vi "BenchC2_DEV_v15_5.vi"() -> ()   [LabVIEW 2016]
uses:
  BERTTA/x64/Debug/BERTTA.dll
panel:
  out "Started:":string
  in  "SHUTDOWN":bool
  in  "MASTER CONTROL":bool
  in  "Tab Control":T1(tab)
  out "Output File":path caption="selected path"
  in  "Browse folder":path=path "C:/Users/shresplab/Desktop" caption="start path"
  in  "Read Seq":bool
  in  "Save Seq":bool
  in  "Configuration file":path caption="Filename"
  in  "OK Button 2":bool
  out "Boolean":bool
  in  "User (initials)":string
  in  "Project name":string
  in  "Description":string
  out "Led11 12":bool
  out "Led11 11":bool
  out "PUMP1":bool
  out "Target amount":dbl format="Target amount:        %#_g"
  out "Scale weight":dbl format="Scale weight:     %#_4g"
  out "Amount now":dbl format="Amount now:      %#_4g"
  out "Flow rate":dbl format="Flow rate:                   %#_4g"
  out "Time to target":dbl format="Time to target:     %<%H:%M:%S>t"
  out "Current step":dbl format="Current step:              %#_g"
  out "Target":dbl format="Target:                %#_4g"
  out "Amount now":dbl format="Amount now:    %#_4g"
  out "Amount now":dbl
  out "Target":dbl
  out "Current step":dbl
  out "Time to target":dbl format="%<%H:%M:%S>t"
  out "Flow rate":dbl
  out "Amount now":dbl
  out "Scale weight":dbl
  out "Target amount":dbl
  out "PUMP2":bool
  out "Sensor OK 6":bool
  out "Sensor OK 5":bool
  out "Sensor OK 4":bool
  out "Sensor OK 3":bool
  in  "OK Button":bool
  in  "Add comment":string
  out "Tr":dbl format="Tr:              %#_4g"
  out "Tj in":dbl format="Tj in:        %#_4g"
  out "Tj out":dbl format="Tj out:        %#_4g"
  out "T set":dbl format="T set:          %#_g"
  out "Current step":i32 format="Current step:  %.0f"
  out "RPM":dbl format="RPM:          %#_g"
  out "Torque 2":dbl format="Torque:      %#_g"
  out "PUMP3":bool
  out "Target amount":dbl
  out "Scale weight":dbl
  out "Amount now":dbl
  out "Flow rate":dbl
  out "Time to target":dbl format="%<%H:%M:%S>t"
  out "Current step":dbl
  out "Target":dbl
  out "Amount now":dbl
  out "Waveform Chart 5":dynamicdata(graph)
  out "Waveform Chart 6":dynamicdata(graph)
  out "Waveform Chart 7":dynamicdata(graph)
  out "Led11 10":bool
  out "T external 3":dbl format="T (S2):       %#_4g"
  out "Table":string[][](table)=[["14.8.2017 18.06.59", "0,000000", "417,670000", "-0,150000", "1,000000", "22,220000", "23,366837", "23,574959", "23,985852", "23,690000", "240,000000", "4,000000", "0,000000", "397,000000", "-397,000000", "1,000000"], ["14.8.2017 18.07.06", "0,000000", "417,640000", "-0,120000", "1,000000", "22,220000", "23,763115", "23,906257", "23,985694", "23,680000", "240,000000", "4,000000", "0,000000", "397,000000", "-397,000000", "1,000000"], ["14.8.2017 18.07.13", "0,000000", "417,640000", "-0,120000", "1,000000", "22,220000", "23,965922", "24,013440", "23,984906", "23,670000", "240,000000", "4,100000", "3,000000", "397,000000", "-397,000000", "1,000000"], ["14.8.2017 18.07.21", "0,000000", "417,640000", "-0,120000", "1,000000", "22,220000", "23,943860", "23,900110", "23,987113", "23,670000", "240,000000", "4,000000", "0,000000", "397,000000", "-397,000000", "1,000000"], ["14.8.2017 18.07.28", "0,000000", "417,640000", "-0,120000", "1,000000", "22,220000", "23,736328", "23,600018", "23,989004", "23,660000", "240,000000", "4,000000", "0,000000", "397,000000", "-397,000000", "1,000000"], ["14.8.2017 18.07.36", "0,000000", "417,640000", "-0,120000", "1,000000", "22,220000", "23,480910", "23,324538", "23,991053", "23,660000", "240,000000", "4,000000", "0,000000", "397,000000", "-397,000000", "1,000000"], ["14.8.2017 18.07.43", "0,000000", "417,640000", "-0,120000", "2,000000", "22,220000", "23,195579", "23,008270", "23,999093", "23,650000", "240,000000", "4,000000", "0,000000", "397,000000", "-397,000000", "1,000000"], ["14.8.2017 18.07.51", "0,000000", "417,650000", "-417,650000", "1,000000", "22,220000", "22,862541", "22,649021", "24,003979", "23,650000", "240,000000", "4,000000", "0,000000", "397,000000", "-397,000000", "2,000000"], ["14.8.2017 18.07.58", "0,000000", "417,640000", "0,010000", "1,000000", "22,220000", "22,541353", "22,354878", "24,005398", "23,650000", "240,000000", "4,000000", "0,000000", "397,000000", "-397,000000", "1,000000"], ["14.8.2017 18.08.06", "0,000000", "417,640000", "0,010000", "1,000000", "22,220000", "22,347931", "22,253738", "24,007605", "23,640000", "240,000000", "4,100000", "0,000000", "397,000000", "-397,000000", "1,000000"], ["14.8.2017 18.08.13", "0,000000", "417,640000", "0,010000", "1,000000", "22,220000", "22,329030", "22,302102", "24,006028", "23,640000", "240,000000", "4,000000", "0,000000", "395,820000", "-395,820000", "1,000000"], ["14.8.2017 18.08.20", "0,000000", "417,640000", "0,010000", "1,000000", "22,220000", "22,466849", "22,511320", "24,002403", "23,630000", "240,000000", "4,000000", "0,000000", "395,830000", "-0,010000", "1,000000"], ["14.8.2017 18.08.28", "0,000000", "417,640000", "0,010000", "1,000000", "22,220000", "22,707062", "22,835101", "24,000984", "23,620000", "240,000000", "4,000000", "0,000000", "395,830000", "-0,010000", "1,000000"], ["14.8.2017 18.08.35", "0,000000", "417,640000", "0,010000", "1,000000", "22,220000", "23,054104", "23,232979", "24,001299", "23,600000", "240,000000", "4,000000", "0,000000", "395,830000", "-0,010000", "1,000000"], ["14.8.2017 18.08.43", "0,000000", "417,640000", "0,010000", "1,000000", "22,220000", "23,412371", "23,522793", "24,002560", "23,590000", "240,000000", "4,000000", "0,000000", "395,820000", "0,000000", "1,000000"], ["14.8.2017 18.08.51", "0,000000", "417,640000", "0,010000", "1,000000", "22,220000", "23,596247", "23,656125", "24,003821", "23,580000", "240,000000", "4,000000", "0,000000", "395,820000", "0,000000", "1,000000"]]
  out "LED_5":bool
  out "LED_4":bool
  in  "PAUSE/RUN 4":bool
  in  "TEMP RAMP":dbl[][](array[numeric])
  out "LED_3":bool
  out "LED_2":bool
  out "LED_1":bool
  out "LED_MANUAL":bool
  in  "Reset 6":bool
  in  "Manual/Ramp":bool=TRUE
  in  "Sensor selector":bool=TRUE
  in  "Tr/Tj mode selector":bool=TRUE
  out "LED STOP":bool
  in  "Failsafe":dbl=20.0 format="Failsafe temperature:            %#_g"
  out "Current temp":dbl format="Current temperature S1:       %#_4g"
  out "Sensor OK":bool
  out "T external 2":dbl format="Current temperature S2:       %#_4g"
  in  "OK Button 3":bool
  out "Waveform Chart":dynamicdata(graph)
  in  "X scale":i64(slide)=50 scale=0.0..100.0
  in  "PAUSE/RUN 9":bool=TRUE
  in  "PAUSE/RUN 8":bool=TRUE
  in  "PAUSE/RUN 7":bool=TRUE
  out "Led11 7":bool
  out "Led11 6":bool
  out "Led11 7":bool
  out "Led11 6":bool
  out "Led5 7":bool
  out "Led4 6":bool
  out "Waveform Chart 18":dynamicdata(graph)
  in  "PAUSE/RUN 3":bool
  in  "Tube select 3":u32(ring) items=["Big tube", "Double big tube", "Medium tube", "Small tube"]
  in  "Reset 8":bool
  out "Led11 9":bool
  in  "?":bool
  in  "Grams / min 3":dbl
  out "RPM 3":dbl format="%_4f"
  out "Flow rate (g/min) 3":dbl
  out "Scale reading 3":dbl
  out "Step amount now 3":dbl
  out "Total amount now 3":dbl
  out "Elapsed / step 3":dbl format="%<%H:%M:%S>t"
  out "Time to target 3":dbl format="%<%H:%M:%S>t"
  out "Led5 5":bool
  out "Led4 5":bool
  out "Led3 5":bool
  out "Led2 5":bool
  out "Led1 5":bool
  in  "PumpSeq 6":dbl[][](array[numeric])=[[0.0, 0.0, 0.0, 0.0, 0.0, 0.0, 0.0, 0.0, 0.0, 0.0], [0.0, 0.0, 0.0, 0.0, 0.0, 0.0, 0.0, 0.0, 0.0, 0.0], [0.0, 0.0, 0.0, 0.0, 0.0, 0.0, 0.0, 0.0, 0.0, 0.0], [0.0, 0.0, 0.0, 0.0, 0.0, 0.0, 0.0, 0.0, 0.0, 0.0], [0.0, 0.0, 0.0, 0.0, 0.0, 0.0, 0.0, 0.0, 0.0, 0.0], [0.0, 0.0, 0.0, 0.0, 0.0, 0.0, 0.0, 0.0, 0.0, 0.0], [0.0, 0.0, 0.0, 0.0, 0.0, 0.0, 0.0, 0.0, 0.0, 0.0], [0.0, 0.0, 0.0, 0.0, 0.0, 0.0, 0.0, 0.0, 0.0, 0.0], [0.0, 0.0, 0.0, 0.0, 0.0, 0.0, 0.0, 0.0, 0.0, 0.0], [0.0, 0.0, 0.0, 0.0, 0.0, 0.0, 0.0, 0.0, 0.0, 0.0]]
  out "Led11 8":bool
  in  "PAUSE/RUN 2":bool
  in  "Tube select 2":u32(ring) items=["Big tube", "Double big tube", "Medium tube", "Small tube"]
  out "Led11 7":bool
  in  "?":bool
  in  "Grams / min 2":dbl
  out "RPM 2":dbl format="%_4f"
  out "Flow rate (g/min) 2":dbl
  out "Scale reading 2":dbl
  out "Step amount now 2":dbl
  out "Total amount now 2":dbl
  out "Elapsed / step 2":dbl format="%<%H:%M:%S>t"
  out "Time to target 2":dbl format="%<%H:%M:%S>t"
  out "Led5 4":bool
  out "Led4 4":bool
  out "Led3 4":bool
  out "Led2 4":bool
  out "Led1 4":bool
  in  "PumpSeq 5":dbl[][](array[numeric])=[[0.0, 0.0, 0.0, 0.0, 0.0, 0.0, 0.0, 0.0, 0.0, 0.0], [0.0, 0.0, 0.0, 0.0, 0.0, 0.0, 0.0, 0.0, 0.0, 0.0], [0.0, 0.0, 0.0, 0.0, 0.0, 0.0, 0.0, 0.0, 0.0, 0.0], [0.0, 0.0, 0.0, 0.0, 0.0, 0.0, 0.0, 0.0, 0.0, 0.0], [0.0, 0.0, 0.0, 0.0, 0.0, 0.0, 0.0, 0.0, 0.0, 0.0], [0.0, 0.0, 0.0, 0.0, 0.0, 0.0, 0.0, 0.0, 0.0, 0.0], [0.0, 0.0, 0.0, 0.0, 0.0, 0.0, 0.0, 0.0, 0.0, 0.0], [0.0, 0.0, 0.0, 0.0, 0.0, 0.0, 0.0, 0.0, 0.0, 0.0], [0.0, 0.0, 0.0, 0.0, 0.0, 0.0, 0.0, 0.0, 0.0, 0.0], [0.0, 0.0, 0.0, 0.0, 0.0, 0.0, 0.0, 0.0, 0.0, 0.0]]
  out "Led11 6":bool
  in  "Reset 7":bool
  in  "PAUSE/RUN":bool
  in  "Tube select":u32(ring) items=["Big tube", "Double big tube", "Medium tube", "Small tube"]
  out "Led11 5":bool
  out "RPM":dbl format="RPM                      %_4f"
  out "Flow rate (g/min)":dbl format="Flow rate               %#_g"
  out "Scale reading":dbl format="Scale reading       %#_g"
  out "Step amount now":dbl format="Step amount       %#_g"
  out "Total amount now":dbl format="Total amount      %#_g"
  out "Elapsed / step":dbl format="Elapsed / step      %<%H:%M:%S>t"
  out "Time to target":dbl format="Time to target     %<%H:%M:%S>t"
  out "Led5 3":bool
  out "Led4 3":bool
  out "Led3 3":bool
  out "Led2 3":bool
  out "Led1 3":bool
  in  "PumpSeq 4":dbl[][](array[numeric])=[[0.0, 0.0, 0.0, 0.0, 0.0, 0.0, 0.0, 0.0, 0.0, 0.0], [0.0, 0.0, 0.0, 0.0, 0.0, 0.0, 0.0, 0.0, 0.0, 0.0], [0.0, 0.0, 0.0, 0.0, 0.0, 0.0, 0.0, 0.0, 0.0, 0.0], [0.0, 0.0, 0.0, 0.0, 0.0, 0.0, 0.0, 0.0, 0.0, 0.0], [0.0, 0.0, 0.0, 0.0, 0.0, 0.0, 0.0, 0.0, 0.0, 0.0], [0.0, 0.0, 0.0, 0.0, 0.0, 0.0, 0.0, 0.0, 0.0, 0.0], [0.0, 0.0, 0.0, 0.0, 0.0, 0.0, 0.0, 0.0, 0.0, 0.0], [0.0, 0.0, 0.0, 0.0, 0.0, 0.0, 0.0, 0.0, 0.0, 0.0], [0.0, 0.0, 0.0, 0.0, 0.0, 0.0, 0.0, 0.0, 0.0, 0.0], [0.0, 0.0, 0.0, 0.0, 0.0, 0.0, 0.0, 0.0, 0.0, 0.0]]
  in  "?":bool
  in  "Grams / min":dbl format="Manual g/min:  %#_g"
  out "Led11 4":bool
  in  "Reset 5":bool
  in  "OK Button 4":bool
  out "Waveform Chart 16":dynamicdata(graph)
  in  "OK Button 5":bool
  out "Waveform Chart 17":dynamicdata(graph)
  in  "OK Button 6":bool
  in  "PAUSE/RUN 5":bool
  in  "?":bool
  in  "Scale port":dbl=5.0
  out "Waveform Chart 15":dynamicdata(graph)
  in  "OK Button 8":bool
  in  "PAUSE/RUN 6":bool
  in  "Set RPM":i32
  in  "Remote / Manual":bool
  out "RPM":dbl
  out "Torque":dbl
  out "Waveform Chart 4":dynamicdata(graph)
  in  "OK Button 7":bool
  in  "CDAQ Temp Control":tag="cDAQ9188XT-1C3BF12Mod1"
  in  "CDAQ PAM Control":tag="cDAQ9188XT-1C3BF12Mod1"
  in  "PORT PUMP2":i32 format="PUMP 2 PORT:  %.0f"
  in  "PORT PUMP3":i32 format="PUMP 3 PORT:  %.0f"
  in  "PORT PUMP1":i32 format="PUMP 1 PORT:  %.0f"
  in  "Save PortDev":bool
  in  "LAUDA":i32 format="LAUDA PORT:  %.0f"
  in  "HEIDOLPH":i32 format="HEIDOLPH PORT:  %.0f"
  in  "SCALE1":i32 format="SCALE 1 PORT:  %.0f"
  in  "SCALE2":i32 format="SCALE 2 PORT:  %.0f"
  in  "SCALE 3":i32 format="SCALE 3 PORT:  %.0f"
  # "PUMP & SCALE 1"
  # "PUMP & SCALE 2"
  # "PUMP & SCALE 3"
  # "STEP"
  # "STEP"
  # "STEP"
  # "TOTAL"
  # "TOTAL"
  # "TOTAL"
  # "Temperature sensor:"
  # "Manual control:"
  # "MANUAL"
  # "RAMP"
  # "Temp Target       Time Target          Wait Time"
  # "STOP"
  # "g              min"
  # "g              min"
  # "g              min"
  # "PAM control"
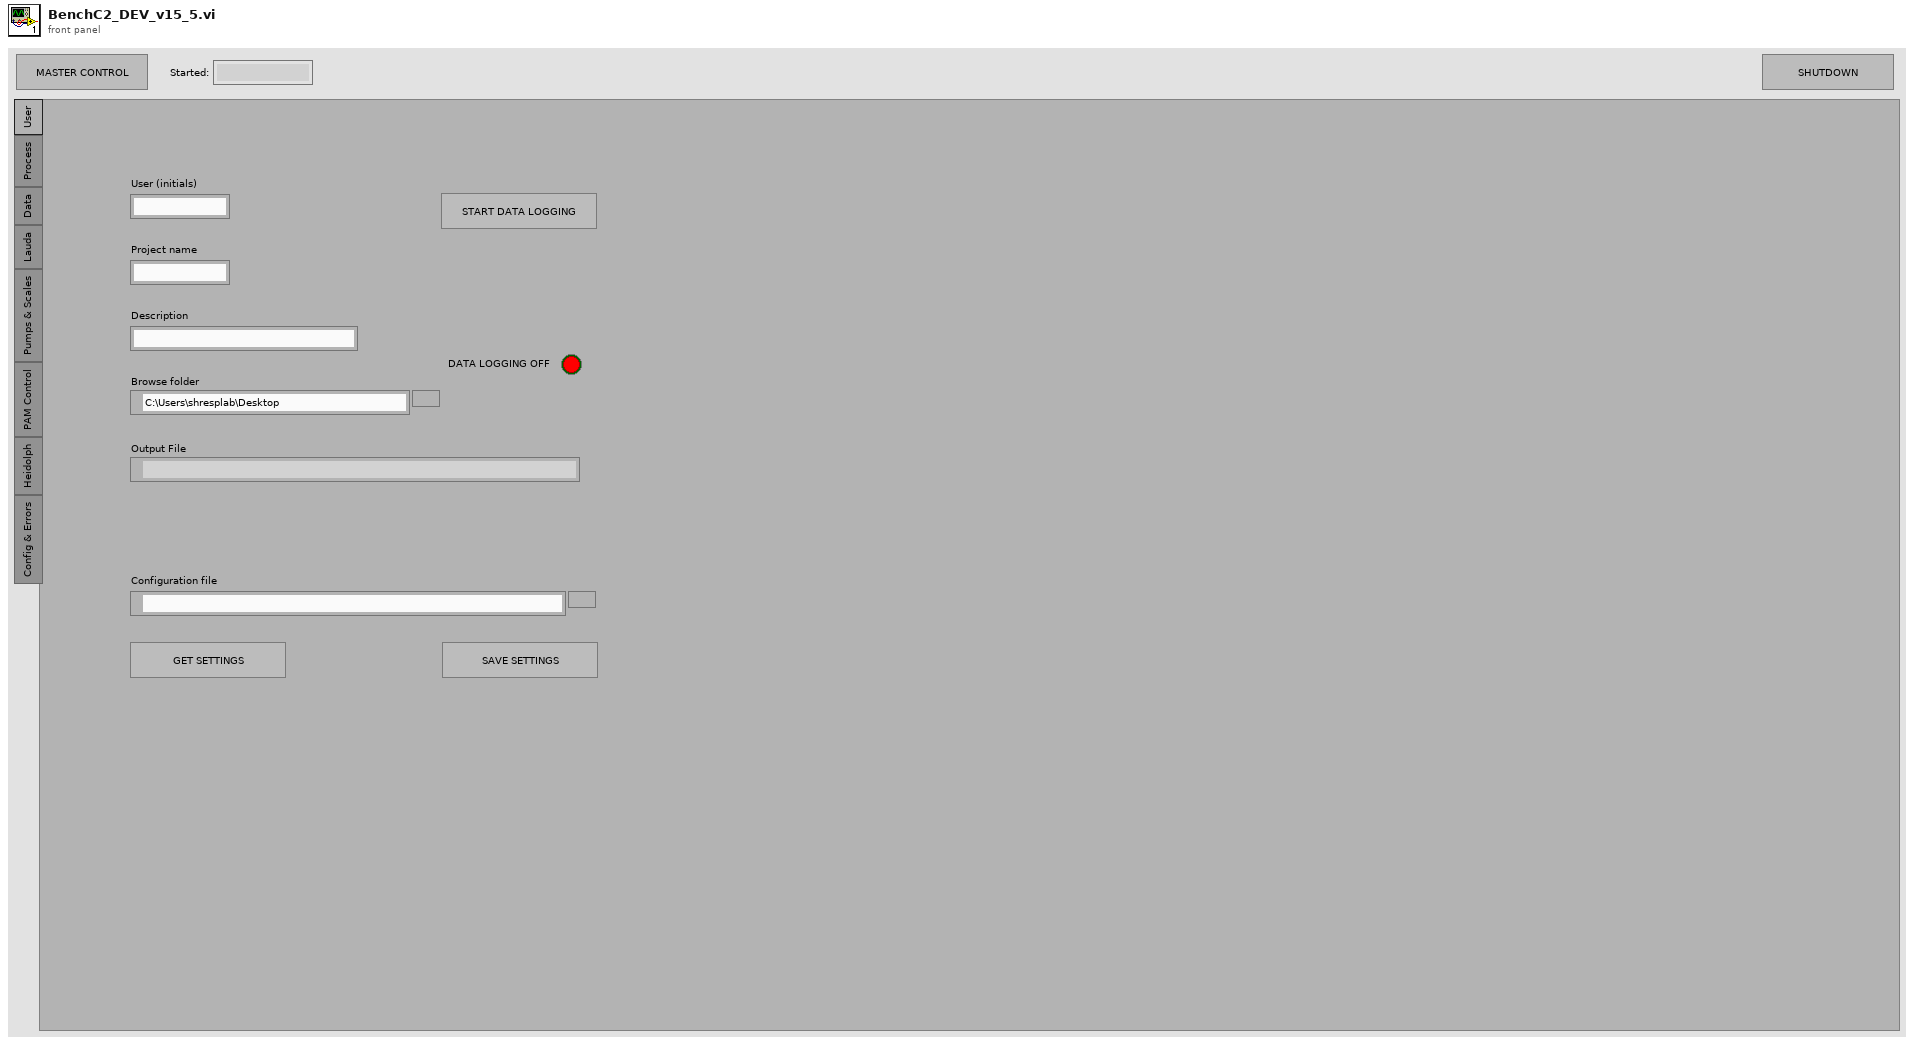
[diagram p1: front panel]
types:
  T1 = enum32{"User", "Process", "Data", "Lauda", "Pumps & Scales", "PAM Control", "Heidolph", "Config & Errors"}
diagram:
  n1 = while {
    i -> [w211]
    stop <- FALSE stop-if-true
    w105 = i64 1000 ("y")
    # "SCALE & PUMP 3"
    n2 = Boolean To (0,1)(Boolean="PAUSE/RUN 7") -> (0, 1=w3:i16)
    n3 = Boolean To (0,1)(Boolean="PAUSE/RUN 8") -> (0, 1=w2:i16)
    n4 = Boolean To (0,1)(Boolean="PAUSE/RUN 9") -> (0, 1=w1:i16)
    n5 = And(x="PAUSE/RUN 6", y="MASTER CONTROL") -> (x .and. y?=w94:bool)
    n6 = feedback #1() -> (w110:dbl[][])  [unwired: 1 in]
    n7 = Select(t="TEMP RAMP", s="Reset 6", f=w110) -> (s? t:f=w111:dbl[][])
    n8 = feedback-in #1(w111) -> ()
    n9 = Initialize Array(0.0 ("element"), 5 ("dimension size"), 3 ("dimension size")) -> (w154:dbl[][])
    n10 = Select(t="Set RPM", s=w94, f=10) -> (s? t:f=w97:i32)
    n11 = Not(x="MASTER CONTROL") -> (.not. x?=w260:bool)
    n12 = Replace Array Subset(array=w154, new element=w110, index (row)=0, index (col)=0 ("disabled index (col)")) -> (w128:dbl[][])
    n13 = control-ref of="This VI"() -> (w90:refnum<vi>)
    n14 = Multiply(x="X scale", y=w105) -> (x*y=w106:i64)
    n15 = Boolean To (0,1)(Boolean=w260) -> (0, 1=w261:i16)
    n16 = Add(x=w106, y=w105) -> (x+y=w101:i64)
    n17 = for {
      N: w261 -> [_]
      n18 = Get Date/Time String(want seconds? (F)=TRUE) -> (time string=→"Started:":string)  [unwired: 2 in, 1 out]
    }
    n19 = feedback #2() -> (w104:i64)  [unwired: 1 in]
    n20 = feedback-in #2(w101) -> ()
    n21 = Boolean To (0,1)(Boolean="Sensor selector") -> (0, 1=w136:i16)
    n22 = Boolean To (0,1)(Boolean="SHUTDOWN") -> (0, 1=w88:i16)
    n23 = call "shutdown sequence.vi"("SHUTDOWN"="SHUTDOWN", "VI in"=w90) -> ()  [unwired: 10 in]
    n24 = Not Equal?(x=w104, y=w101) -> (x != y?=w103:bool)
    n25 = property on="Waveform Chart" class="WFChart (strict)"() -> ("History Data"=w108:dynamicdata[])  [unwired: 2 in, 2 out]
    n26 = Boolean To (0,1)(Boolean=w103) -> (0, 1=w100:i16)
    n27 = Array Size(array=w108) -> (size(s)=w102:i32)
    n28 = Boolean To (0,1)(Boolean="SHUTDOWN") -> (0, 1=w91:i16)
    n29 = Boolean To (0,1)(Boolean="Tr/Tj mode selector") -> (0, 1=w148:i16)
    n30 = formula code="int SensorLED1 = 0, SensorLED0 = 0, ModeLED1 = 0, ModeLED0 = 0;\nif(Sensor==1) SensorLED1 = 1;\nif(Sensor==0) SensorLED0 = 1;\nif(Tr_Tj==1) ModeLED1 = 1;\nif(Tr_Tj==0) ModeLED0 = 1;"("Tr_Tj"=w148, "Sensor"=w136) -> ("SensorLED1"=w146:i32, "SensorLED0"=w144:i32, "ModeLED1"=w129:i32, "ModeLED0"=w139:i32)
    n31 = Equal?(x=w146, y=1.0) -> (x = y?=→"Sensor OK 3":bool)
    n32 = Equal?(x=w144, y=1.0) -> (x = y?=→"Sensor OK 4":bool)
    n33 = for {
      N: w100 -> [_]
      tunnel: w102 -> [w268]
      tunnel: w101 -> [w267]
      n34 = Add(x=w268, y=w267) -> (x+y=w266:i64)
      n35 = property on="Waveform Chart" class="WFChart (strict)"("XScale.Maximum"=w266) -> ()  [unwired: 2 in, 2 out]
    }
    n36 = call "MReadRS232_2.vi"("port1"="LAUDA", "dev1"=1, "enable5"=w3, "port2"="LAUDA", "dev2"=2, "port3"="HEIDOLPH", "enable7"=w1, "enable8"=0, "dev7"=5, "dev8"=0, "port7"="SCALE 3", "port8"=0, "dev5"=5, "enable6"=w2, "port5"="SCALE1", "dev4"=4, "dev6"=5, "port6"="SCALE2", "port4"="HEIDOLPH", "dev3"=3) -> ("params"=w27:dbl[])  [unwired: 6 in, 1 out]
    n37 = call "HEI_CTRL.vi"("shutdown"=w91, "Set RPM"=w97, "Remote / Manual"="Remote / Manual", "port3"="HEIDOLPH") -> ()  [unwired: 8 in]
    n38 = And(x="MASTER CONTROL", y="PAUSE/RUN 4") -> (x .and. y?=w170:bool)
    n39 = Index Array(array=w128, index (col)=2 ("disabled index (col)")) -> (element=w158:dbl[])  [unwired: 1 in]
    n40 = Equal?(x=w129, y=1.0) -> (x = y?=→"Sensor OK 6":bool)
    n41 = Equal?(x=w139, y=1.0) -> (x = y?=→"Sensor OK 5":bool)
    n42 = Boolean To (0,1)(Boolean=w170) -> (0, 1=w169:i16)
    n43 = Boolean To (0,1)(Boolean="Manual/Ramp") -> (0, 1=w171:i16)
    n44 = Boolean To (0,1)(Boolean="Reset 6") -> (0, 1=w173:i16)
    n45 = Build Array("LAUDA", "HEIDOLPH", "SCALE1", "SCALE2", "SCALE 3", "PORT PUMP1", "PORT PUMP2", "PORT PUMP3") -> (w115:i32[])
    n46 = Index Array(array=w128, index (col)=1 ("disabled index (col)")) -> (element=w160:dbl[])  [unwired: 1 in]
    n47 = Index Array(array=w128, index (col)=0 ("disabled index (col)")) -> (element=w161:dbl[])  [unwired: 1 in]
    n48 = call "LaudaDAQ.vi"("device name"="CDAQ Temp Control") -> (1:"Tj out"=→"Tj out":dbl, "data"=w248:dynamicdata, "Sensor OK"=→"Sensor OK":bool, 4:"Tj out"=→"Tj in":dbl, "T external 2"=w93:dbl)  [unwired: 5 in, 1 out]
    "T external 2" <- w93
    "T external 3" <- w93
    n49 = call "Ramp_Lauda_v3.vi"("manual"=w171, "Tr_Tj"=w148, "shutdown"=w88, "S1_S2"=w136, "Tr"=w27, "T_fail"="Failsafe", "enable"=w169, "time_set"=w160, "reset"=w173, "time_wait"=w158, "T_S2"=w93, "port"="LAUDA", "T_sp"=w161) -> ("LED_1"=→"LED_1":bool, "LED_manual"=→"LED_MANUAL":bool, "LED_2"=→"LED_2":bool, "step"=w126:dbl, "LED_stop"=→"LED STOP":bool, "LED_3"=→"LED_3":bool, "LED 4"=→"LED_4":bool, "LED 5"=→"LED_5":bool, "setpoint"=w123:dbl, "Tr_out"=w168:dbl, "T int"=w167:dbl)  [unwired: 2 in, 2 out]
    "Tr" <- w168
    "T set" <- w123
    "Current temp" <- w168
    n50 = Boolean To (0,1)(Boolean="Save PortDev") -> (0, 1=w214:i16)
    n51 = for {
      N: w214 -> [_]
      tunnel: w115 -> [w314]
      tunnel: "Save PortDev" -> [w315]
      n52 = call "Convert to Dynamic Data"("Array"=w314) -> ("Dynamic Data Type"=w313:dynamicdata)  [unwired: 3 in]
      n53 = call "Write To Measurement File3"("Signals"=w313, "Reset"=w315) -> ()  [unwired: 15 in, 3 out]
    }
    n54 = Add(x=w126, y=1.0) -> (x+y=→"Current step":dbl)
    n55 = Less?(x=w211, y=1.0) -> (x < y?=w209:bool)
    n56 = Index Array(array=w27, index=3) -> (element=w202:dbl)
    "RPM" <- w202
    "RPM" <- w202
    n57 = Index Array(array=w27, index=2) -> (element=w204:dbl)
    n58 = Boolean To (0,1)(Boolean=w209) -> (0, 1=w210:i16)
    n59 = Divide(x=w204, y=10.0) -> (x/y=w201:dbl)
    "Torque" <- w201
    "Torque 2" <- w201
    n60 = for {
      N: w210 -> [_]
      tunnel: w209 -> [w308]
      n61 = while {
        tunnel: [w311] -> w307
        tunnel: w308 -> [w309]
        stop <- w312 stop-if-true
        n62 = call "Read From Measurement File2"("Enable"=TRUE, "Reset"=w309) -> ("Signals"=w311:dynamicdata, "EOF?"=w312:bool)  [unwired: 4 in, 4 out]
      }
      n63 = call "Convert from Dynamic Data2"("Dynamic Data Type"=w307) -> ("Array"=w293:dbl[])  [unwired: 3 in]
      n64 = Index Array(array=w293, index=0) -> (element=w300:dbl)
      n65 = Index Array(array=w293, index=1) -> (element=w299:dbl)
      n66 = Index Array(array=w293, index=2) -> (element=w298:dbl)
      n67 = Index Array(array=w293, index=3) -> (element=w297:dbl)
      n68 = Index Array(array=w293, index=4) -> (element=w296:dbl)
      n69 = Index Array(array=w293, index=5) -> (element=w290:dbl)
      n70 = Index Array(array=w293, index=6) -> (element=w292:dbl)
      n71 = Index Array(array=w293, index=7) -> (element=w291:dbl)
      n72 = property on="LAUDA" class="DigNum (strict)"("Val(Sgnl)"=w300) -> ()  [unwired: 2 in, 2 out]
      n73 = property on="HEIDOLPH" class="DigNum (strict)"("Val(Sgnl)"=w299) -> ()  [unwired: 2 in, 2 out]
      n74 = property on="SCALE1" class="DigNum (strict)"("Val(Sgnl)"=w298) -> ()  [unwired: 2 in, 2 out]
      n75 = property on="SCALE2" class="DigNum (strict)"("Val(Sgnl)"=w297) -> ()  [unwired: 2 in, 2 out]
      n76 = property on="SCALE 3" class="DigNum (strict)"("Val(Sgnl)"=w296) -> ()  [unwired: 2 in, 2 out]
      n77 = property on="PORT PUMP2" class="DigNum (strict)"("Val(Sgnl)"=w292) -> ()  [unwired: 2 in, 2 out]
      n78 = property on="PORT PUMP3" class="DigNum (strict)"("Val(Sgnl)"=w291) -> ()  [unwired: 2 in, 2 out]
      n79 = property on="PORT PUMP1" class="DigNum (strict)"("Val(Sgnl)"=w290) -> ()  [unwired: 2 in, 2 out]
    }
    n80 = Merge Signals(w202, w201) -> (w200:dynamicdata)
    "Waveform Chart 4" <- w200
    "Waveform Chart 6" <- w200
    n81 = Boolean To (0,1)(Boolean="OK Button 3") -> (0, 1=w229:i16)
    n82 = for {
      N: w229 -> [_]
      n83 = property on="Waveform Chart" class="WFChart (strict)"("History Data"=dynamicdata[] []) -> ()  [unwired: 2 in, 2 out]
    }
    n84 = Merge Signals(w123, w168, w167, w248) -> (w249:dynamicdata)
    "Waveform Chart" <- w249
    "Waveform Chart 5" <- w249
    n85 = Boolean To (0,1)(Boolean="OK Button 4") -> (0, 1=w227:i16)
    n86 = for {
      N: w227 -> [_]
      n87 = property on="Waveform Chart 18" class="WFChart (strict)"("History Data"=dynamicdata[] []) -> ()  [unwired: 2 in, 2 out]
    }
    n88 = call "IsmaCTRL.vi"("FR_manual"="Grams / min", "tube selector"="Tube select", "Manual"="?", "Reset"="Reset 5", "Pause"="PAUSE/RUN", "Setpoint_W   /   Setpoint_T"="PumpSeq 4", "Enable"="MASTER CONTROL", "Scale"=w27) -> ("Boolean 9"=→"Led11 5" →"Led11 10":bool, "Boolean"=→"Led1 3":bool, "Boolean 2"=→"Led2 3":bool, "Total target"=→"Target":dbl, "Boolean 3"=→"Led3 3":bool, "Boolean 4"=→"Led4 3":bool, "lastAmount"=→"Step amount now":dbl, "step"=→"Current step":dbl, "Boolean 5"=→"Led5 3":bool, "Boolean 6"=→"Led4 6":bool, "Boolean 7"=→"Led5 7":bool, "FR"=w70:dbl, "RPM"=w62:dbl, "Weight"=w66:dbl, "elapsed"=→"Elapsed / step":dbl, "time_to_target"=→"Time to target" →"Time to target":dbl, "pumpCTRL"=w82:dbl, "Target_step"=→"Target amount":dbl, "Boolean 8"=w74:bool)  [unwired: 1 out]
    "Flow rate" <- w70
    "Scale weight" <- w66
    "Led11 4" <- w74
    "Scale reading" <- w66
    "Flow rate (g/min)" <- w70
    "RPM" <- w62
    n89 = Boolean To (0,1)(Boolean="OK Button 5") -> (0, 1=w134:i16)
    n90 = for {
      N: w134 -> [_]
      n91 = property on="Waveform Chart 16" class="WFChart (strict)"("History Data"=dynamicdata[] []) -> ()  [unwired: 2 in, 2 out]
    }
    n92 = Multiply(x=w66, y=-1.0 ("x")) -> (x*y=→"Amount now" →"Amount now" →"Total amount now":dbl)
    n93 = Greater?(x=w82, y=70.0) -> (0:→"PUMP1":bool)
    n94 = Boolean To (0,1)(Boolean="OK Button 6") -> (0, 1=w132:i16)
    n95 = And(x="PAUSE/RUN", y=w74) -> (x .and. y?=w190:bool)
    n96 = Merge Signals(w66, w70) -> (w135:dynamicdata)
    "Waveform Chart 18" <- w135
    n97 = for {
      N: w132 -> [_]
      n98 = property on="Waveform Chart 17" class="WFChart (strict)"("History Data"=dynamicdata[] []) -> ()  [unwired: 2 in, 2 out]
    }
    n99 = feedback #3() -> (w191:bool)  [unwired: 1 in]
    n100 = feedback-in #3(w190) -> ()
    n101 = Not Equal?(x=w191, y=w190) -> (x != y?=w189:bool)
    n102 = Boolean To (0,1)(Boolean=w189) -> (0, 1=w188:i16)
    n103 = for {
      N: w188 -> [_]
      n104 = property on="PAUSE/RUN" class="Bool (strict)"("Val(Sgnl)"=FALSE ("Value (Signaling)")) -> ()  [unwired: 2 in, 2 out]
    }
    n105 = Boolean To (0,1)(Boolean="OK Button 7") -> (0, 1=w225:i16)
    n106 = for {
      N: w225 -> [_]
      n107 = property on="Waveform Chart 4" class="WFChart (strict)"("History Data"=dynamicdata[] []) -> ()  [unwired: 2 in, 2 out]
    }
    n108 = Boolean To (0,1)(Boolean="OK Button 8") -> (0, 1=w197:i16)
    n109 = call "IsmaCTRL_2.vi"("FR_manual"="Grams / min 2", "tube selector"="Tube select 2", "Manual"="?", "Reset"="Reset 7", "Pause"="PAUSE/RUN 2", "Setpoint_W   /   Setpoint_T"="PumpSeq 5", "Enable"="MASTER CONTROL", "Scale"=w27) -> ("Boolean 9"=→"Led11 7" →"Led11 11":bool, "Boolean"=→"Led1 4":bool, "Boolean 2"=→"Led2 4":bool, "Total target"=→"Target":dbl, "Boolean 3"=→"Led3 4":bool, "Boolean 4"=→"Led4 4":bool, "lastAmount"=→"Amount now" →"Step amount now 2":dbl, "step"=→"Current step":dbl, "Boolean 5"=→"Led5 4":bool, "Boolean 6"=→"Led11 6":bool, "Boolean 7"=→"Led11 7":bool, "FR"=w51:dbl, "RPM"=w53:dbl, "Weight"=w52:dbl, "elapsed"=→"Elapsed / step 2":dbl, "time_to_target"=→"Time to target" →"Time to target 2":dbl, "pumpCTRL"=w45:dbl, "Target_step"=→"Target amount":dbl, "Boolean 8"=w35:bool)  [unwired: 1 out]
    "Scale weight" <- w52
    "Flow rate" <- w51
    "Led11 6" <- w35
    "Scale reading 2" <- w52
    "Flow rate (g/min) 2" <- w51
    "RPM 2" <- w53
    n110 = for {
      N: w197 -> [_]
      n111 = property on="Waveform Chart 15" class="WFChart (strict)"("History Data"=dynamicdata[] []) -> ()  [unwired: 2 in, 2 out]
    }
    n112 = Merge Signals(w52, w51) -> (w185:dynamicdata)
    "Waveform Chart 16" <- w185
    n113 = Multiply(x=w52, y=-1.0) -> (x*y=→"Amount now" →"Total amount now 2":dbl)
    n114 = And(x="PAUSE/RUN 2", y=w35) -> (x .and. y?=w183:bool)
    n115 = Greater?(x=w45, y=70.0) -> (0:→"PUMP2":bool)
    n116 = feedback #4() -> (w184:bool)  [unwired: 1 in]
    n117 = feedback-in #4(w183) -> ()
    n118 = Not Equal?(x=w184, y=w183) -> (x != y?=w182:bool)
    n119 = Boolean To (0,1)(Boolean=w182) -> (0, 1=w181:i16)
    n120 = for {
      N: w181 -> [_]
      n121 = property on="PAUSE/RUN 2" class="Bool (strict)"("Val(Sgnl)"=FALSE ("Value (Signaling)")) -> ()  [unwired: 2 in, 2 out]
    }
    n122 = call "IsmaCTRL_3.vi"("FR_manual"="Grams / min 3", "tube selector"="Tube select 3", "Manual"="?", "Reset"="Reset 8", "Pause"="PAUSE/RUN 3", "Setpoint_W   /   Setpoint_T"="PumpSeq 6", "Enable"="MASTER CONTROL", "Scale"=w27) -> ("Boolean 9"=→"Led11 9" →"Led11 12":bool, "Boolean"=→"Led1 5":bool, "Boolean 2"=→"Led2 5":bool, "Total target"=→"Target":dbl, "Boolean 3"=→"Led3 5":bool, "Boolean 4"=→"Led4 5":bool, "lastAmount"=→"Amount now" →"Step amount now 3":dbl, "step"=→"Current step":dbl, "Boolean 5"=→"Led5 5":bool, "Boolean 6"=→"Led11 6":bool, "Boolean 7"=→"Led11 7":bool, "FR"=w19:dbl, "RPM"=w17:dbl, "Weight"=w18:dbl, "elapsed"=→"Elapsed / step 3":dbl, "time_to_target"=→"Time to target" →"Time to target 3":dbl, "pumpCTRL"=w24:dbl, "Target_step"=→"Target amount":dbl, "Boolean 8"=w8:bool)  [unwired: 1 out]
    "Scale weight" <- w18
    "Flow rate" <- w19
    "Led11 8" <- w8
    "Scale reading 3" <- w18
    "Flow rate (g/min) 3" <- w19
    "RPM 3" <- w17
    n123 = call "MWriteRS232_2.vi"("PORT PUMP3"="PORT PUMP3", "PORT PUMP2"="PORT PUMP2", "PORT PUMP1"="PORT PUMP1", "PORT LAUDA"="LAUDA", "enable3"=w2, "enable4"=w1, "enable2"=w3, "P3"=w17, "P2"=w53, "P1"=w62, "LAUDA"=w123) -> ()  [unwired: 1 in]
    n124 = Multiply(x=w18, y=-1.0) -> (x*y=→"Amount now" →"Total amount now 3":dbl)
    n125 = Greater?(x=w24, y=70.0) -> (0:→"PUMP3":bool)
    n126 = And(x="MASTER CONTROL", y=w8) -> (x .and. y?=w176:bool)
    n127 = Merge Signals(w18, w19) -> (w178:dynamicdata)
    "Waveform Chart 17" <- w178
    n128 = feedback #5() -> (w177:bool)  [unwired: 1 in]
    n129 = feedback-in #5(w176) -> ()
    n130 = Not Equal?(x=w177, y=w176) -> (x != y?=w175:bool)
    n131 = Boolean To (0,1)(Boolean=w175) -> (0, 1=w174:i16)
    n132 = for {
      N: w174 -> [_]
      n133 = property on="PAUSE/RUN 3" class="Bool (strict)"("Val(Sgnl)"=FALSE ("Value (Signaling)")) -> ()  [unwired: 2 in, 2 out]
    }
    n134 = call "Convert to Dynamic Data4"("2D Array"="PumpSeq 6") -> ("Dynamic Data Type"=w235:dynamicdata)  [unwired: 3 in]
    n135 = call "Convert to Dynamic Data3"("2D Array"="PumpSeq 5") -> ("Dynamic Data Type"=w236:dynamicdata)  [unwired: 3 in]
    n136 = call "Convert to Dynamic Data2"("2D Array"="PumpSeq 4") -> ("Dynamic Data Type"=w238:dynamicdata)  [unwired: 3 in]
    n137 = Merge Signals(w235, w236, w238) -> (w237:dynamicdata)
    n138 = Boolean To (0,1)(Boolean="Save Seq") -> (0, 1=w234:i16)
    n139 = for {
      N: w234 -> [_]
      tunnel: w237 -> [w356]
      tunnel: "Configuration file" -> [w357]
      tunnel: "Save Seq" -> [w355]
      n140 = call "Write To Measurement File2"("Signals"=w356, "Reset"=w355, "Filename"=w357) -> ()  [unwired: 14 in, 3 out]
    }
    n141 = Merge Signals(w135, w185, w178) -> (w250:dynamicdata)
    n142 = Merge Signals(w66, w52, w18) -> (→"Waveform Chart 7":dynamicdata)
    n143 = Boolean To (0,1)(Boolean="Read Seq") -> (0, 1=w233:i16)
    n144 = for {
      N: w233 -> [_]
      tunnel: "Configuration file" -> [w330]
      tunnel: "Read Seq" -> [w329]
      n145 = while {
        tunnel: [w354] -> w350
        tunnel: w330 -> [w353]
        tunnel: w329 -> [w351]
        stop <- w352 stop-if-true
        n146 = call "Read From Measurement File"("Filename"=w353, "Reset"=w351) -> ("Signals"=w354:dynamicdata, "EOF?"=w352:bool)  [unwired: 4 in, 4 out]
      }
      n147 = call "Convert from Dynamic Data"("Dynamic Data Type"=w350) -> ("Array"=w342:dbl[][])  [unwired: 3 in]
      n148 = Array Subset(array=w342, index (row)=20 ("index"), length (row)=10 ("length")) -> (w347:dbl[][])  [unwired: 2 in]
      n149 = Array Subset(array=w342, index (row)=10 ("index"), length (row)=10 ("length")) -> ()  [unwired: 2 in, 1 out]
      n150 = Array Subset(array=w342, index (row)=0 ("index"), length (row)=10 ("length")) -> ()  [unwired: 2 in, 1 out]
      n151 = Array Subset(array=w342, index (row)=30 ("index"), length (row)=8 ("length")) -> (w331:dbl[][])  [unwired: 2 in]
      n152 = property on="PumpSeq 4" class="Arr (strict)"("Val(Sgnl)"=w347) -> ()  [unwired: 2 in, 2 out]
      n153 = Index Array(array=w331, index (row)=2, index (col)=0 ("disabled index (col)")) -> ()  [unwired: 1 out]
      n154 = Index Array(array=w331, index (row)=4, index (col)=0 ("disabled index (col)")) -> ()  [unwired: 1 out]
      n155 = Index Array(array=w331, index (row)=0, index (col)=1 ("disabled index (col)")) -> ()  [unwired: 1 out]
      n156 = Index Array(array=w331, index (row)=1, index (col)=1 ("disabled index (col)")) -> ()  [unwired: 1 out]
    }
    n157 = Merge Signals(w249, w250, w200) -> (w207:dynamicdata)
    n158 = call "Build Table"("Include time data"=TRUE, "Signals"=w207) -> ("Table"=w257:string[][])  [unwired: 3 in, 6 out]
    n159 = Boolean To (0,1)(Boolean="PAUSE/RUN 5") -> (0, 1=w150:i16)
    n160 = for {
      N: w150 -> [_]
      tunnel: "MASTER CONTROL" -> [w272]
      tunnel: "PAUSE/RUN 5" -> [w271]
      n161 = And(x=w271, y="?") -> (x .and. y?=w280:bool)
      n162 = dll-call lib="C:/Users/shresplab/OneDrive - Kemira Oyj/Documents/GitHub/Bertta/BERTTA/x64/Debug/BERTTA.dll" fn="mettler"("port"="Scale port", "msg"=1) -> ("return type"=w274:dbl)  [unwired: 5 in, 2 out]
      n163 = And(x=w272, y=w280) -> (x .and. y?=w277:bool)
      n164 = Initialize Array(FALSE, 1 ("dimension size")) -> (w279:bool[])
      n165 = Replace Array Subset(array=w279, new element=w277, index=0) -> (w276:bool[])
      n166 = call "Convert to Dynamic Data5"("Double"=w274) -> ("Dynamic Data Type"=→"Waveform Chart 15":dynamicdata)  [unwired: 3 in]
      n167 = call "DAQ Assistant"("data"=w276, "device name"="CDAQ PAM Control") -> ()  [unwired: 16 in, 2 out]
    }
    n168 = Delete From Array(array=w257, length=13, index (col)=0 ("index (row)")) -> (array with subset deleted=→"Table":string[][])  [unwired: 1 in, 1 out]
    n169 = call "filenameparser_09.vi"("Description"="Description", "start path"="Browse folder", "Project name"="Project name", "User (initials)"="User (initials)", "OK Button in"="OK Button 2") -> ("appended path 2"=w223:path, "appended path"=w253:path)  [unwired: 4 in, 1 out]
    "Output File" <- w223
    n170 = Boolean To (0,1)(Boolean="OK Button") -> (0, 1=w252:i16)
    n171 = for {
      N: w252 -> [_]
      tunnel: w253 -> [w321]
      w325 = " " ("string")
      n172 = property on="Add comment" class="Str"("Val(Sgnl)"="" ("Value (Signaling)")) -> ()  [unwired: 2 in, 2 out]
      n173 = Get Date/Time String(want seconds? (F)=TRUE) -> (date string=w328:string, time string=w326:string)  [unwired: 2 in]
      n174 = Concatenate Strings(w328, w325, w326, w325, "Add comment") -> (w324:string)
      n175 = feedback #6() -> (w323:string[])  [unwired: 1 in]
      n176 = Build Array (concatenate)(w323, w324) -> (w322:string[])
      n177 = feedback-in #6(w322) -> ()
      n178 = Write to Text File(file (use dialog)=w321, text=w322) -> ()  [unwired: 2 in, 3 out]
    }
    n179 = call "Header Names 4.vi"("Dynamic Data"=w207) -> ("Signals Out"=w208:dynamicdata)  [unwired: 10 in]
    n180 = call "Write To Measurement File"("Signals"=w208, "Enable"="OK Button 2", "Filename"=w223) -> ()  [unwired: 14 in, 3 out]
    "Boolean" <- "OK Button 2"
  }
